vi "numerical-integration-test1-callback.vi"(9 "U":T1, 10 "X":T1, 11 "Info":variant) -> (0 "Error":bool, 3 "XDOT":T1)   [LabVIEW 2019]
uses:
  <vilib>/Analysis/Matrix/Datatypes/RealMatrix.ctl
  <vilib>/Rock Robotics/WPI/ThirdParty/JAS_Junk/TrajLib/MatBuilder_Create.vi
  <vilib>/Rock Robotics/WPI/ThirdParty/JAS_Junk/TrajLib/Trajectory_Library.lvlib
  <vilib>/Analysis/Matrix/NI_Matrix.lvlib
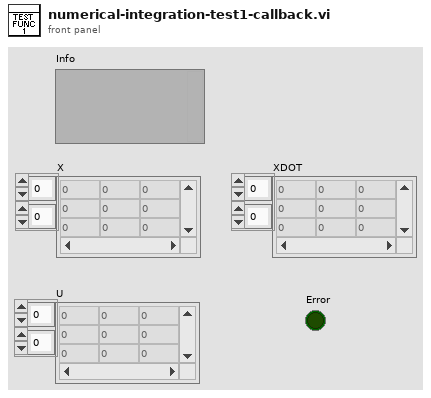
[diagram p1: front panel]
types:
  T1 = typedef "NI_Matrix.lvlib/RealMatrix.ctl" = dbl[][]
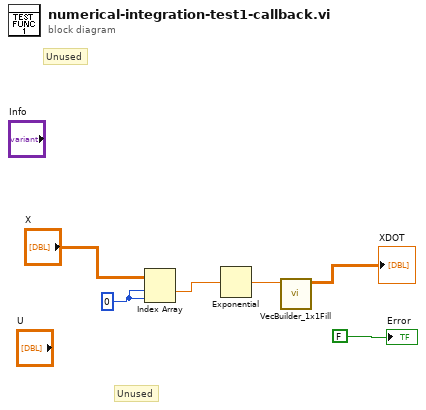
[diagram p0: block diagram]
diagram:
  w3 = 0 ("index (row)")
  # "Unused"
  # "Unused"
  n1 = Index Array(array="X", index (row)=w3, index (col)=w3) -> (element=w4:dbl)
  n2 = Exponential(1:w4) -> (0:w5:dbl)
  n3 = call <vilib>:"VecBuilder_1x1Fill.vi"("R0_C0"=w5) -> ("output matrix"=→"XDOT":T1)  [unwired: 10 in]
  "Error" <- FALSE ("Error")
